vi "Autonomous Independent.vi"() -> ()   [LabVIEW 2019]
doc: "This VI is called when autonomous begins, and will automatically be terminated when autonomous ends. You can carry out timed or sensor driven robot movement independently without needing to return to the caller."
uses:
  JoysticksGlobal.vi
  MotorsGlobal.vi
  <vilib>/Rock Robotics/Network Tables/NT Read String.vi
panel:
  in  "EnableAuto":bool
  out "Over?":bool
  in  "Range":cluster{"output high":dbl, "output low":dbl}={"output high"=0.95, "output low"=-0.4} {"output low" format="%.2f"; "output high" format="%.2f"}
  in  "Gains":T1={"proportional gain (Kc)"=1.0, "integral time (Ti, min)"=0.01, "derivative time (Td, min)"=0.0} {"derivative time (Td, min)" format="%.3f"; "integral time (Ti, min)" format="%.3f"; "proportional gain (Kc)" format="%.3f"}
  in  "Distance":dbl
  # "Be sure to right-click and choose Data Operations>>Make Current Value default if you want to save the array values with the VI"
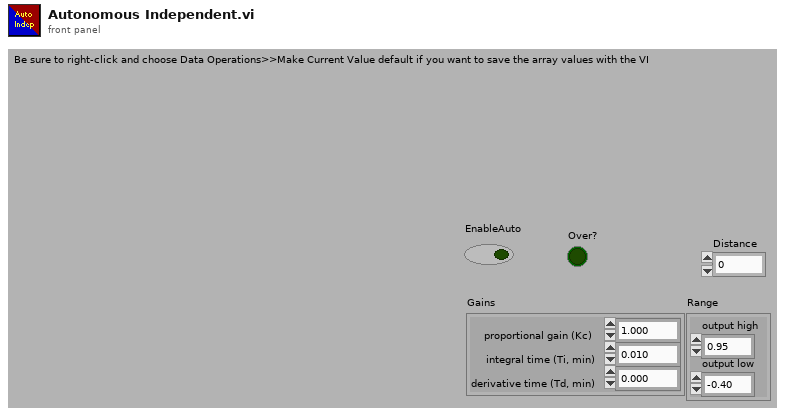
[diagram p1: front panel]
types:
  T1 = cluster{"proportional gain (Kc)":dbl, "integral time (Ti, min)":dbl, "derivative time (Td, min)":dbl}
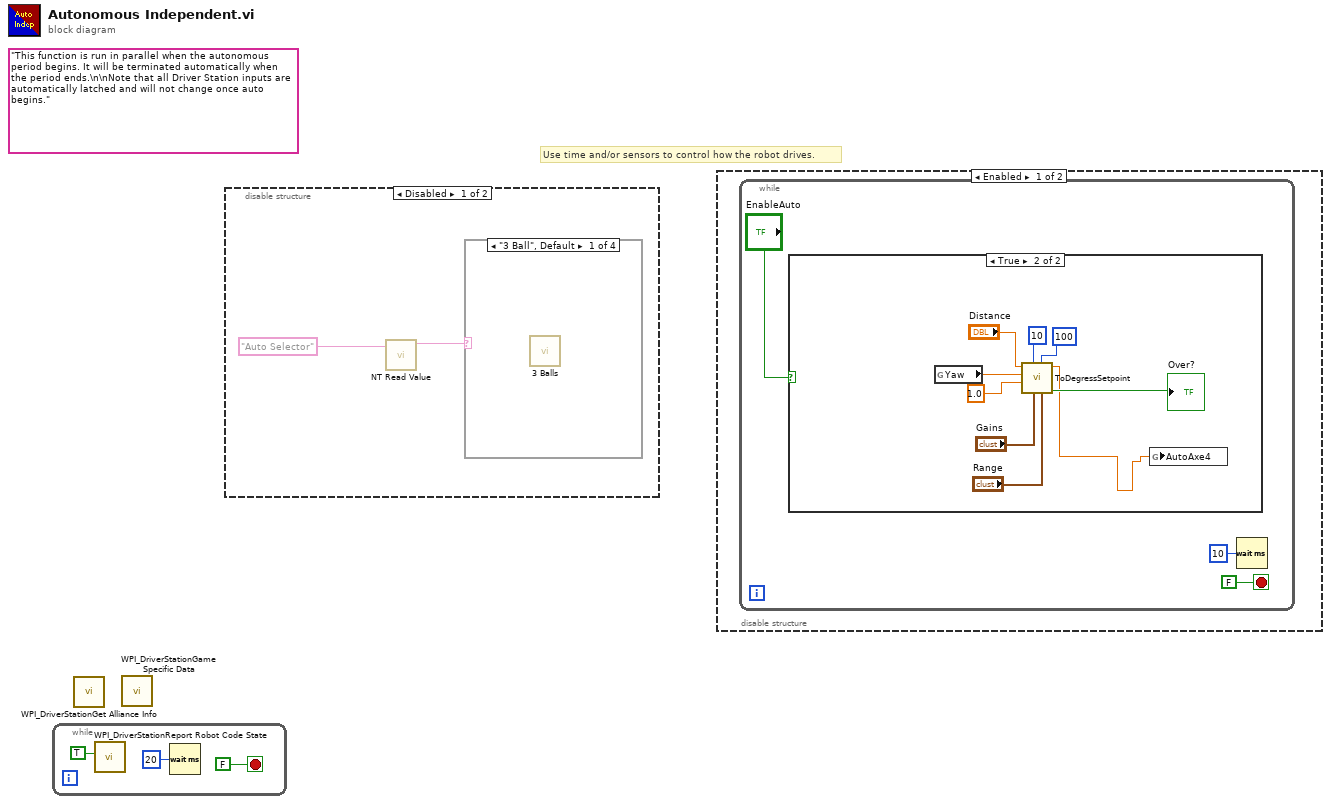
[diagram p0: block diagram]
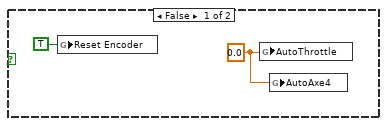
[diagram p2: hidden frame]
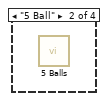
[diagram p4: hidden frame]
diagram:
  (unwired) "This function is run in parallel when the autonomous period begins. It will be terminated automatically when the period ends.\n\nNote that all Driver Station inputs are automatically latched and will not change once auto begins."
  # "Use time and/or sensors to control how the robot drives."
  n1 = while {
    stop <- FALSE stop-if-true
    n2 = call <vilib>:"WPI_DriverStationReport Robot Code State.vi"("Autonomous"=TRUE) -> ()  [unwired: 10 in, 1 out]
    n3 = Wait (ms)(milliseconds to wait=u32 20) -> ()  [unwired: 1 out]
  }
  n4 = call <vilib>:"WPI_DriverStationGet Alliance Info.vi"() -> ()  [unwired: 12 out]
  n5 = call <vilib>:"WPI_DriverStationGame Specific Data.vi"() -> ()  [unwired: 11 in, 1 out]
  n6 = disable-structure shown="Disabled" {
    frame Disabled {
      n7 = call-poly <vilib>:"NT Read Value.vi"("Name"="Auto Selector") -> ("String"=w4:string)  [unwired: 9 in, 1 out]
      n8 = case shown="\"3 Ball\", Default" w4 {
        frame "3 Ball", Default {
          n9 = call "3 Balls.vi"() -> ()  [unwired: 12 in]
        }
        frame "5 Ball" {
          n10 = call "5 Balls.vi"() -> ()  [unwired: 12 in]
        }
        frame "8 Ball" {
        }
        frame "10 Ball" {
        }
      }
    }
    frame Enabled {
    }
  }
  n11 = disable-structure shown="Enabled" {
    frame Enabled {
      n12 = while {
        stop <- FALSE stop-if-true
        n13 = case shown="True" "EnableAuto" {
          frame False {
            w9 = 0.0 ("AutoThrottle")
            n14 = global write "MotorsGlobal.vi" "Reset Encoder"(TRUE ("Reset Encoder")) -> ()
            n15 = global write "JoysticksGlobal.vi" "AutoThrottle"(w9) -> ()
            n16 = global write "JoysticksGlobal.vi" "AutoAxe4"(w9) -> ()
          }
          frame True {
            n17 = global read "MotorsGlobal.vi" "Yaw"() -> (w18:dbl)
            n18 = call "ToDegressSetpoint.vi"("Range"="Range", "Delay After"=100, "Gains"="Gains", "Loop Wait Delay"=10, "Precision"=1.0, "Yaw"=w18, "Setpoint (degress)"="Distance") -> ("Finished?"=→"Over?":bool, "Output"=w11:dbl)  [unwired: 3 in]
            n19 = global write "JoysticksGlobal.vi" "AutoAxe4"(w11) -> ()
          }
        }
        n20 = Wait (ms)(milliseconds to wait=u32 10) -> ()  [unwired: 1 out]
      }
    }
    frame Disabled {
    }
  }
